vi "Cache.Result.Find.vi"(7 "Idx":i32, 8 "error in (no error)":errorcluster, 9 "Serial":string, 10 "Variant":string) -> (0 "error out":errorcluster, 1 "Found?":bool, 2 "File":path)   [LabVIEW 2016]
uses:
  Global/ApplicationGlobal.vi
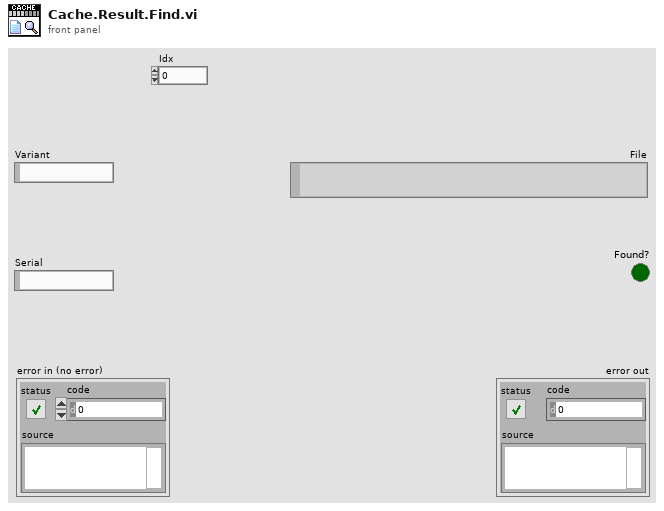
[diagram p1: front panel]
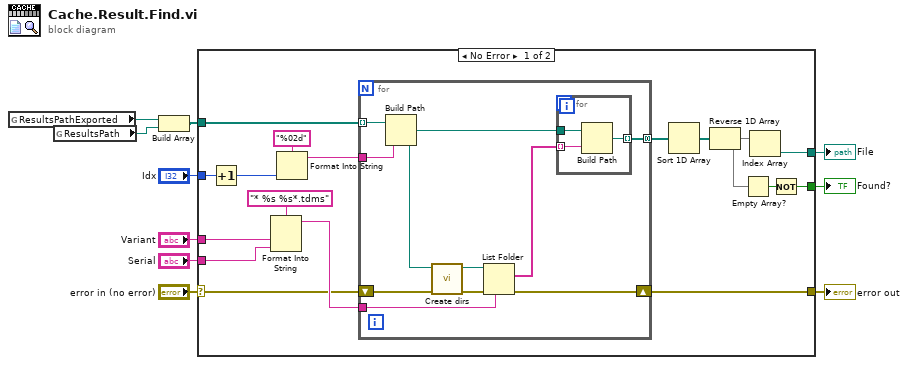
[diagram p0: block diagram]
diagram:
  n1 = global read "ApplicationGlobal.vi" "ResultsPathExported"() -> (w5:path)
  n2 = global read "ApplicationGlobal.vi" "ResultsPath"() -> (w4:path)
  n3 = Build Array(w5, w4) -> (w3:path[])
  n4 = case shown="No Error" "error in (no error)" {
    selector: "error in (no error)" -> [w20 w40]
    tunnel: [w27 w40] -> w10
    tunnel: "Variant" -> [w24 _]
    tunnel: "Serial" -> [w23 _]
    tunnel: [w11 _] -> w6
    tunnel: w3 -> [w22 _]
    tunnel: "Idx" -> [w25 _]
    tunnel: [w15 _] -> w1
    frame No Error {
      n5 = Increment(x=w25) -> (x+1=w14:i32)
      n6 = Format Into String(format string="* %s %s*.tdms" ("pattern"), w24, w23) -> (resulting string=w21:string)  [unwired: 2 in, 1 out]
      n7 = Format Into String(format string="%02d", w14) -> (resulting string=w12:string)  [unwired: 2 in, 1 out]
      n8 = for {
        tunnel: w21 -> [w34]
        tunnel: w22 -> [w33] mode=indexing
        tunnel: [w35] -> w19 mode=concatenating
        shift-right: [w36] -> w27
        shift-left: w20 -> [w29]
        tunnel: w12 -> [w32]
        n9 = Build Path(base path=w33, name or relative path=w32) -> (appended path=w28:path)
        n10 = call "Create dirs.vi"("error in (no error)"=w29, "deepest dir"=w28) -> ("error"=w30:errorcluster)  [unwired: 9 in]
        n11 = List Folder(path=w28, pattern=w34, error in=w30) -> (filenames=w31:string[], error out=w36:errorcluster)  [unwired: 1 in, 2 out]
        n12 = for {
          tunnel: [w39] -> w35 mode=indexing
          tunnel: w28 -> [w37]
          tunnel: w31 -> [w38] mode=indexing
          n13 = Build Path(base path=w37, name or relative path=w38) -> (appended path=w39:path)
        }
      }
      n14 = Sort 1D Array(array=w19) -> (sorted array=w18:path[])
      n15 = Reverse 1D Array(array=w18) -> (reversed array=w17:path[])
      n16 = Empty Array?(array=w17) -> (empty?=w16:bool)
      n17 = Index Array(array=w17) -> (element=w11:path)  [unwired: 1 in]
      n18 = Not(x=w16) -> (.not. x?=w15:bool)
    }
    frame Error {
    }
  }
  "error out" <- w10
  "File" <- w6
  "Found?" <- w1
